vi "Open Connection.vi"(8 "Error In (no error)":errorcluster, 10 "DB Connection String/Path":string, 11 "DB Operator In":refnum<class "DB Operator.lvclass">) -> (0 "Error Out":errorcluster, 3 "DB Operator Out":refnum<class "DB Operator.lvclass">)   [LabVIEW 2023, in "DB Operator.lvclass"]
uses:
  DB Operator.lvclass
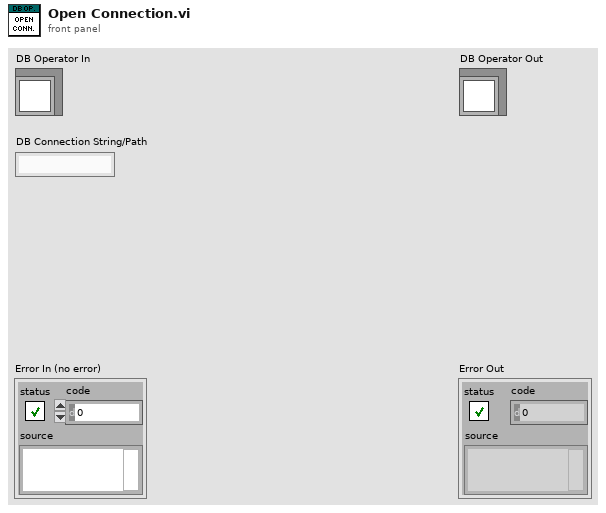
[diagram p1: front panel]
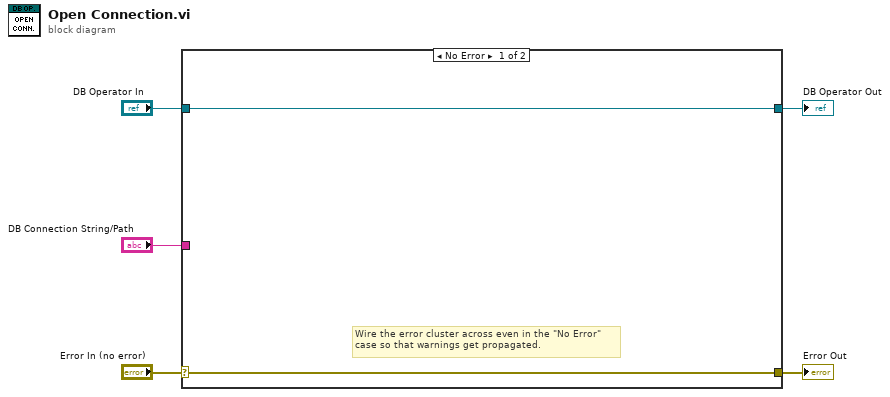
[diagram p0: block diagram]
diagram:
  n1 = case shown="No Error" "Error In (no error)" {
    selector: "Error In (no error)" -> [w6 w9]
    tunnel: [w6 w9] -> w4
    tunnel: [w7 w8] -> w2
    tunnel: "DB Operator In" -> [w7 w8]
    tunnel: "DB Connection String/Path" -> [_ _]
    frame No Error {
      # "Wire the error cluster across even in the \"No Error\"\ncase so that warnings get propagated."
    }
    frame Error {
    }
  }
  "Error Out" <- w4
  "DB Operator Out" <- w2
